vi "FinalSystem.vi"() -> ()   [LabVIEW 2020]
panel:
  in  "VISA resource name":refnum<visa-resource-name>
  in  "Table Control":string[][](table)
  out "Humidity":dbl(graph)
  out "Temperature":dbl(graph)
  out "Humidity":dbl(knob) scale=0.0..100.0
  out "Temperature":dbl(slide) scale=0.0..50.0
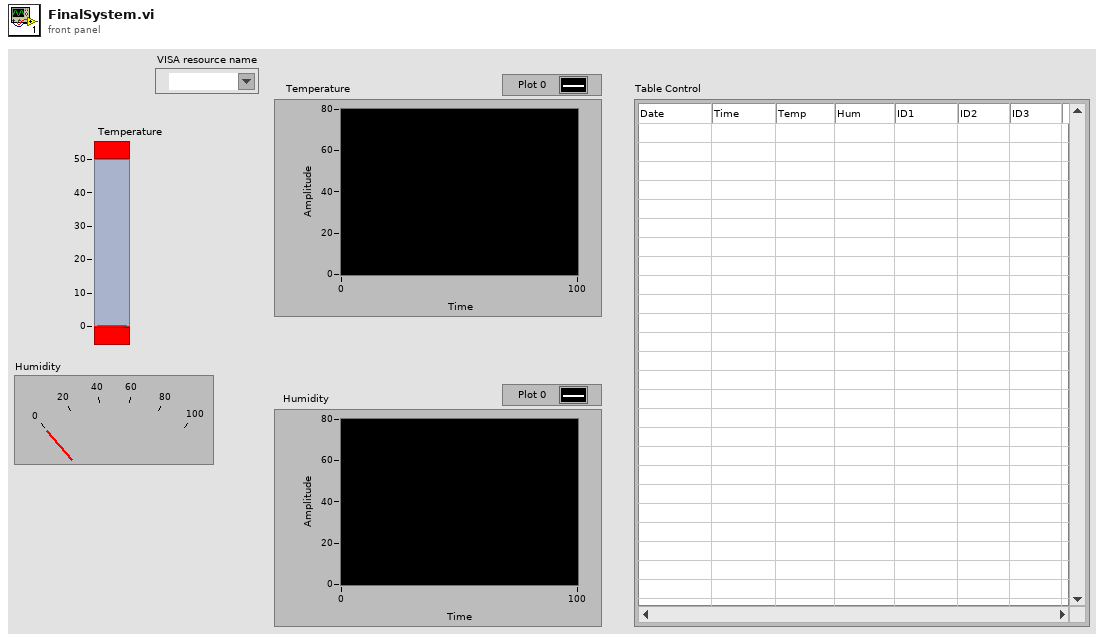
[diagram p1: front panel]
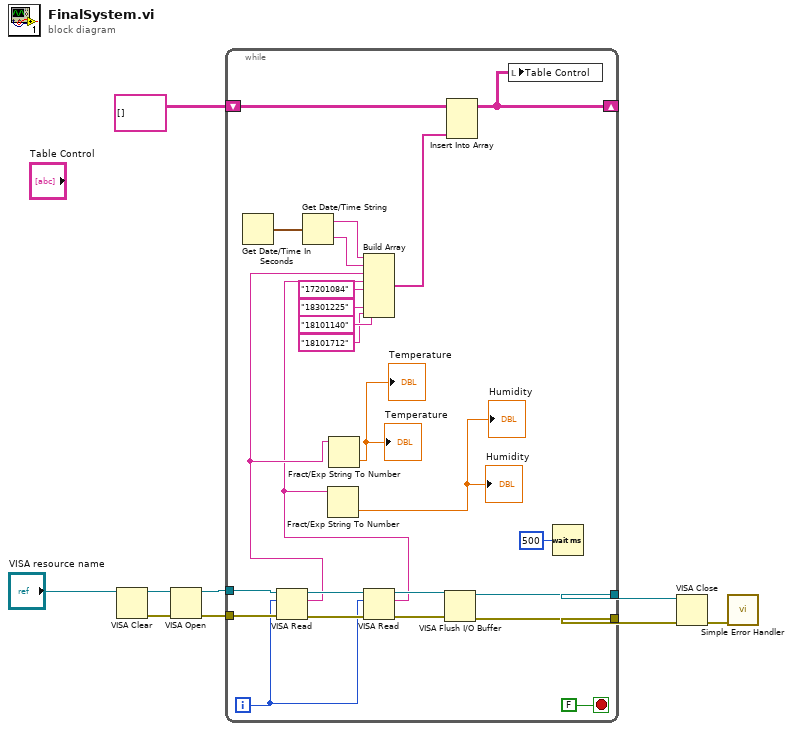
[diagram p0: block diagram]
diagram:
  n1 = VISA Clear(VISA resource name="VISA resource name") -> (VISA resource name out=w8:refnum<visa-resource-name>, error out=w9:errorcluster)  [unwired: 1 in]
  n2 = VISA Open(error in (no error)=w9, VISA resource name=w8) -> (VISA resource name=w6:refnum<visa-resource-name>, error out=w5:errorcluster)  [unwired: 3 in]
  n3 = while {
    tunnel: w6 -> [w34]
    tunnel: w5 -> [w33]
    tunnel: [w28] -> w4
    tunnel: [w27] -> w3
    shift-right: [w23] -> _
    shift-left: string[][] [] -> [w24]
    i -> [w26]
    stop <- FALSE stop-if-true
    n4 = Get Date/Time In Seconds() -> (seconds since 1Jan1904=w20:timestamp)
    n5 = VISA Read(VISA resource name=w34, byte count=w26, error in (no error)=w33) -> (VISA resource name out=w32:refnum<visa-resource-name>, read buffer=w17:string, error out=w31:errorcluster)  [unwired: 1 out]
    n6 = Get Date/Time String(seconds (now)=w20) -> (date string=w19:string, time string=w18:string)  [unwired: 2 in]
    n7 = Fract/Exp String To Number(string=w17) -> (number=→"Temperature" →"Temperature":dbl)  [unwired: 3 in, 1 out]
    n8 = VISA Read(VISA resource name=w32, byte count=w26, error in (no error)=w31) -> (VISA resource name out=w30:refnum<visa-resource-name>, read buffer=w16:string, error out=w29:errorcluster)  [unwired: 1 out]
    n9 = Fract/Exp String To Number(string=w16) -> (number=→"Humidity" →"Humidity":dbl)  [unwired: 3 in, 1 out]
    n10 = Build Array(w19, w18, w17, w16, "17201084" ("element"), "18301225" ("element"), "18101140" ("element"), "18101712" ("element")) -> (w12:string[])
    n11 = VISA Flush I/O Buffer(VISA resource name=w30, error in (no error)=w29) -> (VISA resource name out=w28:refnum<visa-resource-name>, error out=w27:errorcluster)  [unwired: 1 in]
    n12 = Insert Into Array(array=w24, new element=w12) -> (w23:string[][])  [unwired: 2 in]
    n13 = local write "Table Control"(w23) -> ()
    n14 = Wait (ms)(milliseconds to wait=u32 500) -> ()  [unwired: 1 out]
  }
  n15 = VISA Close(VISA resource name=w4, error in (no error)=w3) -> (error out=w7:errorcluster)
  n16 = call <vilib>:"Simple Error Handler.vi"("error in (no error)"=w7) -> ()  [unwired: 4 in, 5 out]
